vi "file names extension handler.vi"(0 "exclude1":string, 1 "File name header":string="BaCrO_CCR", 2 "File name extension":string=".txt", 5 "exclude2":string, 9 "include 1":string="12\n", 11 "include 2":string="2") -> (4 "filtered  numbers":string[](array[string])=["002", "003", "004", "005", "006", "007", "008", "009", "010", "011", "012"], 12 "filetered file names":string[](array[string])=["bacro_ccr.002", "bacro_ccr.003", "bacro_ccr.004", "bacro_ccr.005", "bacro_ccr.006", "bacro_ccr.007", "bacro_ccr.008", "bacro_ccr.009", "bacro_ccr.010", "bacro_ccr.011", "bacro_ccr.012"], 13 "excluded file names":string[](array[string])=["bacro_ccr.000"], 15 "filtered file name no ext":string[](array[string]))   [LabVIEW 2020]
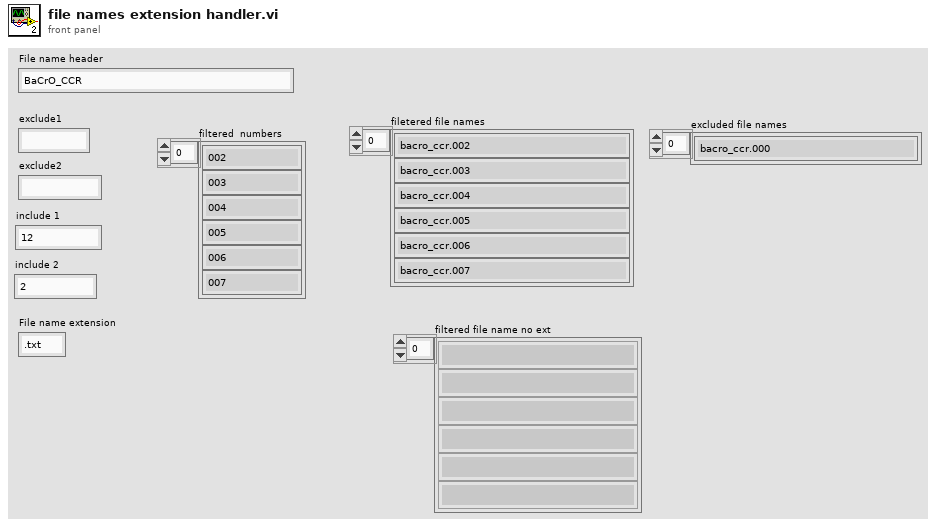
[diagram p1: front panel]
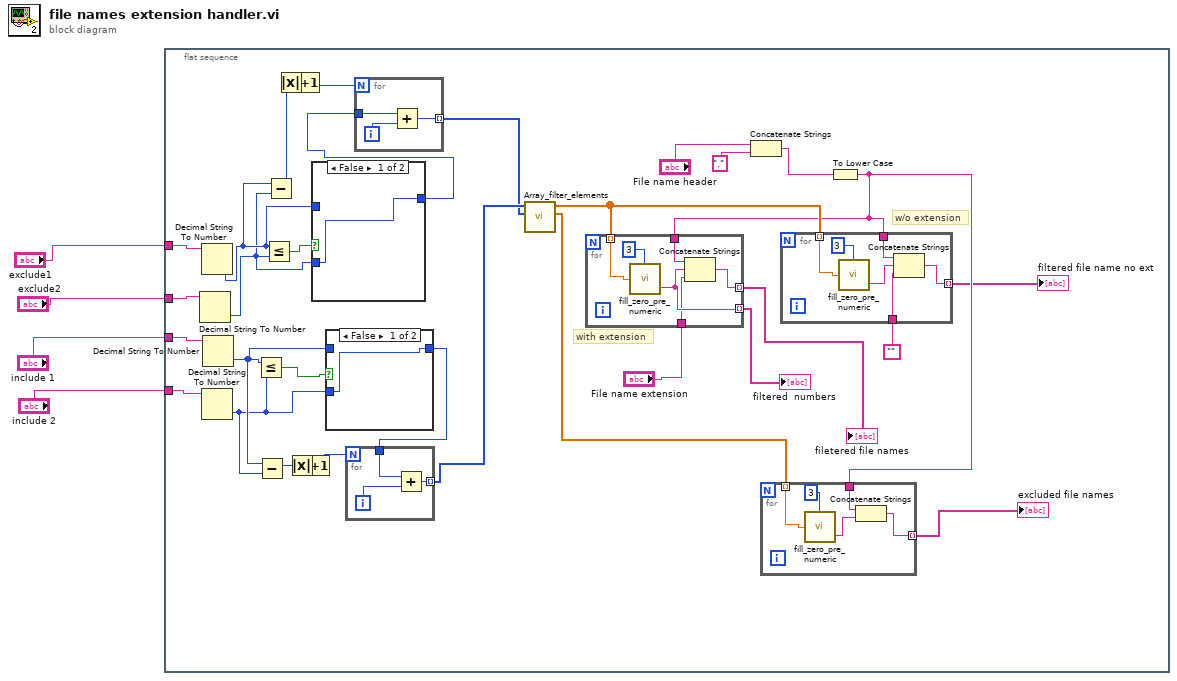
[diagram p0: block diagram]
diagram:
  n1 = flat-sequence {
    tunnel: "include 1" -> [w36]
    tunnel: "include 2" -> [w35]
    tunnel: "exclude1" -> [w34]
    tunnel: "exclude2" -> [w33]
    frame #0 {
      # "w/o extension"
      # "with extension"
      n2 = Decimal String To Number(string=w33) -> (number=w21:i32)  [unwired: 2 in, 1 out]
      n3 = Decimal String To Number(string=w34) -> (number=w22:i32)  [unwired: 2 in, 1 out]
      n4 = Decimal String To Number(string=w35) -> (number=w23:i32)  [unwired: 2 in, 1 out]
      n5 = Decimal String To Number(string=w36) -> (number=w25:i32)  [unwired: 2 in, 1 out]
      n6 = Less Or Equal?(x=w25, y=w23) -> (x <= y?=w32:bool)
      n7 = Subtract(x=w25, y=w23) -> (x-y=w28:i32)
      n8 = Less Or Equal?(x=w22, y=w21) -> (x <= y?=w31:bool)
      n9 = Subtract(x=w22, y=w21) -> (x-y=w30:i32)
      n10 = Absolute Value(x=w30) -> (abs(x)=w29:i32)
      n11 = Absolute Value(x=w28) -> (abs(x)=w27:i32)
      n12 = Increment(x=w29) -> (x+1=w19:i32)
      n13 = Increment(x=w27) -> (x+1=w20:i32)
      n14 = case shown="False" w31 {
        tunnel: [w60 w61] -> w26
        tunnel: w22 -> [_ w61]
        tunnel: w21 -> [w60 _]
        frame False {
        }
        frame True {
        }
      }
      n15 = case shown="False" w32 {
        tunnel: w25 -> [_ w63]
        tunnel: [w62 w63] -> w24
        tunnel: w23 -> [w62 _]
        frame False {
        }
        frame True {
        }
      }
      n16 = for {
        N: w20 -> [_]
        tunnel: w24 -> [w56]
        tunnel: [w54] -> w18 mode=indexing
        i -> [w55]
        n17 = Add(x=w56, y=w55) -> (x+y=w54:i32)
      }
      n18 = for {
        N: w19 -> [_]
        tunnel: w26 -> [w58]
        tunnel: [w57] -> w17 mode=indexing
        i -> [w59]
        n19 = Add(x=w58, y=w59) -> (x+y=w57:i32)
      }
      n20 = call "Array_filter_elements.vi"("smaller set"=w17, "larger set"=w18) -> ("deleted"=w13:dbl[], "filtered"=w9:dbl[])  [unwired: 7 in, 1 out]
      n21 = Concatenate Strings("File name header", "." ("string")) -> (w15:string)
      n22 = To Lower Case(string=w15) -> (all lower case string=w8:string)
      n23 = for {
        tunnel: w9 -> [w48] mode=indexing
        tunnel: [w45] -> w14 mode=indexing
        tunnel: w8 -> [w46]
        tunnel: [w44] -> w11 mode=indexing
        tunnel: "File name extension" -> [w43]
        n24 = call "fill_zero_pre_numeric.vi"("Numeric"=w48, "digit number"=u8 3) -> ("concatenated string"=w44:string)
        n25 = Concatenate Strings(w46, w44, w43) -> (w45:string)
      }
      "filetered file names" <- w14
      "filtered  numbers" <- w11
      n26 = for {
        tunnel: w13 -> [w53] mode=indexing
        tunnel: [w49] -> w12 mode=indexing
        tunnel: w8 -> [w51]
        n27 = call "fill_zero_pre_numeric.vi"("Numeric"=w53, "digit number"=u8 3) -> ("concatenated string"=w50:string)
        n28 = Concatenate Strings(w51, w50) -> (w49:string)
      }
      "excluded file names" <- w12
      n29 = for {
        tunnel: w9 -> [w42] mode=indexing
        tunnel: [w39] -> w5 mode=indexing
        tunnel: w8 -> [w40]
        tunnel: "" -> [w37]
        n30 = call "fill_zero_pre_numeric.vi"("Numeric"=w42, "digit number"=u8 3) -> ("concatenated string"=w38:string)
        n31 = Concatenate Strings(w40, w38, w37) -> (w39:string)
      }
      "filtered file name no ext" <- w5
    }
  }
